vi "Actor Core.vi"(8 "error in":errorcluster, 11 "State in":refnum<class "System Actor.lvclass">) -> (0 "error out":errorcluster, 3 "Actor out":refnum<class "Actor.lvclass">)   [LabVIEW 2014, in "Robot Actor Framework.lvlib" / "System Actor.lvlib" / "System Actor.lvclass"]
doc: "(<B>Filename</B>: Actor Framework.lvlib:Actor.lvclass:Actor Core.vi)\n\nThis override invokes Entry.vi on the initial state, prior to calling the parent Actor Core. Adding this behavior to Actor Core (instead of an override of Pre Launch Init.vi) allows the initial state to launch a nested actor as part of its entry behavior.\n\nReceives messages to the actor, reacts to them, and initiates any error handling that may shut the actor down.\n\nDescendant classes may override this VI to append parallel tasks for the actor to complete while it handles messages. Overrides use the Call Parent Method node."
uses:
  System Actor.lvclass
  <vilib>/ActorFramework/Actor/Actor.lvclass
  System State.ctl
  Command Actor/Command Actor Class/Command State.ctl
  Command Actor/Command Actor Class/Command States.ctl
  Command Processor Actor/Command Processor Actor Class/Command Processor State.ctl
  Command Processor Actor/Command Processor Actor Class/Command Processor States.ctl
  System Actor.lvclass/System Actor.ctl
  Command Processor Actor/States/No Command/No Command.lvclass
  Command Actor/Command Actor Class/Command Actor.lvclass
  Command Processor Actor/Command Processor Actor Class/Command Processor Actor.lvclass
panel:
  out "System Status":T1 {"Command Processor Status"."Commands Behind" scale=0.0..10.0; "Command Processor Status"."Queued Commands" scale=0.0..100.0}
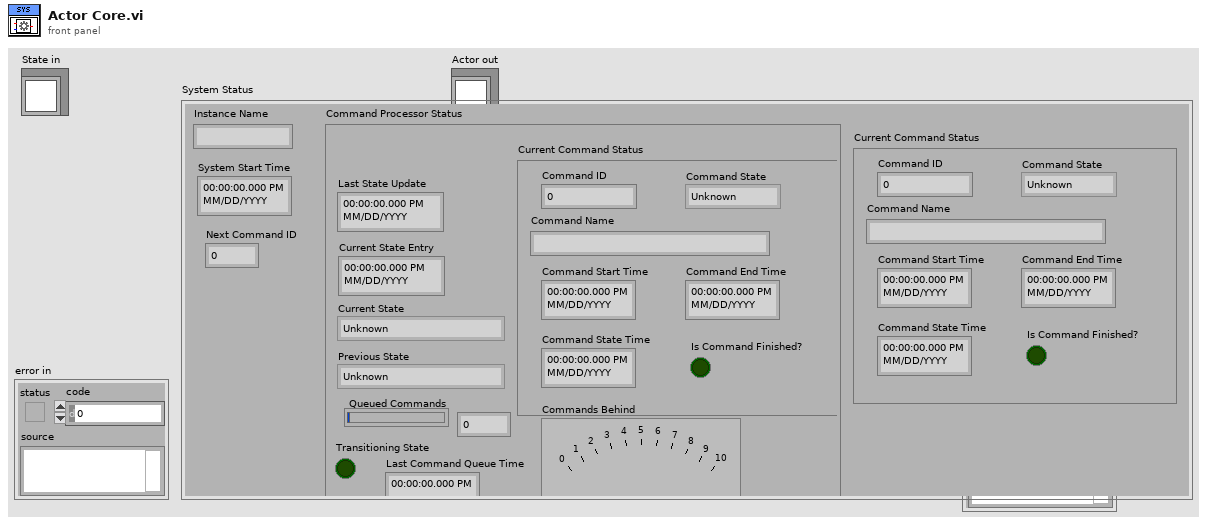
[diagram p1: front panel]
types:
  T1 = typedef "Robot Actor Framework.lvlib/System Actor.lvlib/System Actor.lvclass/System State.ctl" = cluster{"Instance Name":string, "Current Command Status":T2, "System Start Time":timestamp, "Next Command ID":dbl, "Command Processor Status":T4}
  T2 = typedef "Robot Actor Framework.lvlib/Command Actor.lvlib/Command Actor.lvclass/Command State.ctl" = cluster{"Command Name":string, "Command Start Time":timestamp, "Command End Time":timestamp, "Is Command Finished?":bool, "Command ID":u32, "Command State":T3, "Command State Time":timestamp}
  T3 = typedef "Robot Actor Framework.lvlib/Command Actor.lvlib/Command Actor.lvclass/Command States.ctl" = enum16{"Unknown", "Started", "Stopped", "Finished"}
  T4 = typedef "Robot Actor Framework.lvlib/Command Processor Actor.lvlib/Command Processor Actor.lvclass/Command Processor State.ctl" = cluster{"Current State":T5, "Last State Update":timestamp, "Queued Commands":u32, "Current Command Status":T2, "Previous State":T5, "Current State Entry":timestamp, "Transitioning State":bool, "Commands Behind":dbl, "Last Command Queue Time":timestamp}
  T5 = typedef "Robot Actor Framework.lvlib/Command Processor Actor.lvlib/Command Processor Actor.lvclass/Command Processor States.ctl" = enum16{"Unknown", "No Command", "Running Command", "Starting Command", "Stopping Command", "Finishing Command"}
  T6 = enum16{"Critical", "Error", "Warning", "Informational", "Debug"}
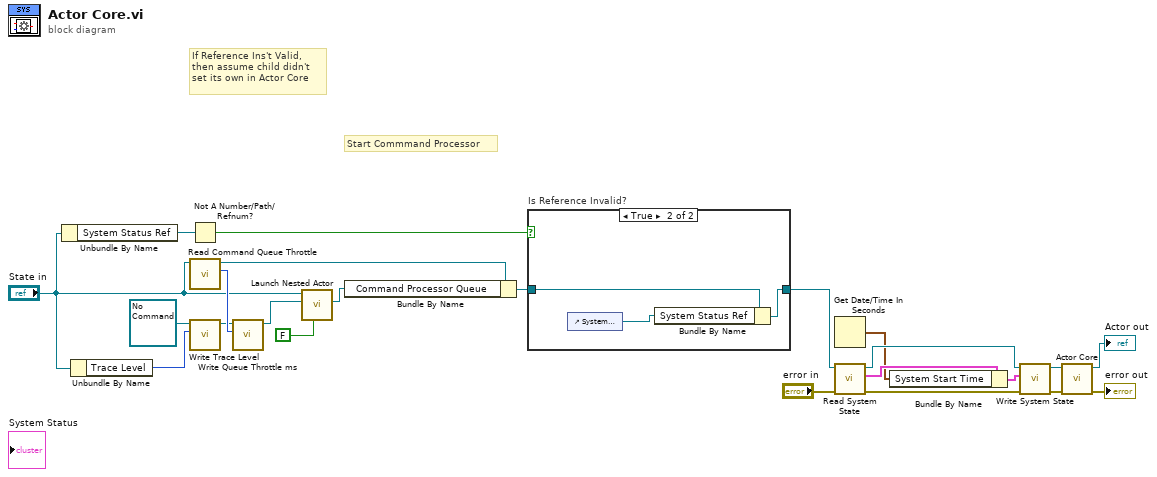
[diagram p0: block diagram]
diagram:
  # "Start Commmand Processor"
  # "If Reference Ins't Valid,\nthen assume child didn't \nset its own in Actor Core"
  n1 = Unbundle By Name("State in") -> ("System Status Ref"=w21:refnum<vi>)
  n2 = Unbundle By Name("State in") -> ("Trace Level"=w1:T6)
  n3 = Not A Number/Path/Refnum?(number/path/refnum=w21) -> (NaN/Path/Refnum?=w20:bool)
  n4 = call-dynamic "Read Command Queue Throttle.vi"("System Actor in"="State in") -> ("Command Queue Throttle ms"=w6:u32, "System Actor out"=w5:refnum<class "System Actor.lvclass">)  [unwired: 8 in, 1 out]
  n5 = call-dynamic "Write Trace Level.vi"("Trace Level"=w1, "Command Processor Actor in"=refnum<class "No Command.lvclass"> refnum ("Robot Actors.lvlib:Command Processor.lvlib:No Command.lvclass")) -> ("Command Processor Actor out"=w2:refnum<class "No Command.lvclass">)  [unwired: 8 in, 1 out]
  n6 = call-dynamic "Write Queue Throttle ms.vi"("Queue Throttle ms"=w6, "Command Processor Actor in"=w2) -> ("Command Processor Actor out"=w7:refnum<class "No Command.lvclass">)  [unwired: 8 in, 1 out]
  n7 = call <vilib>:"Launch Nested Actor.vi"("Open Actor Core front panel? (F)"=FALSE, "Nested Actor"=w7, "Caller Actor in"="State in") -> ("Nested Actor's Enqueuer"=w10:refnum<class "Message Enqueuer.lvclass">)  [unwired: 6 in, 2 out]
  n8 = Bundle By Name(cluster=w5, "Command Processor Queue"=w10) -> (w12:refnum<class "System Actor.lvclass">)
  n9 = case "Is Reference Invalid?" shown="True" w20 {
    tunnel: w12 -> [w24 w27]
    tunnel: [w24 w26] -> w19
    frame False {
    }
    frame True {
      n10 = control-ref of="System Status"() -> (w25:refnum<vi>)
      n11 = Bundle By Name(cluster=w27, "System Status Ref"=w25) -> (w26:refnum<class "System Actor.lvclass">)
    }
  }
  n12 = Get Date/Time In Seconds() -> (seconds since 1Jan1904=w15:timestamp)
  n13 = call-dynamic "Read System State.vi"("error in (no error)"="error in", "System Actor in"=w19) -> ("error out"=w13:errorcluster, "System Status"=w17:T1, "System Actor out"=w18:refnum<class "System Actor.lvclass">)  [unwired: 7 in]
  n14 = Bundle By Name(cluster=w17, "System Start Time"=w15) -> (w16:T1)
  n15 = call-dynamic "Write System State.vi"("error in (no error)"=w13, "System Status"=w16, "System Actor in"=w18) -> ("error out"=w8:errorcluster, "System Actor out"=w9:refnum<class "System Actor.lvclass">)  [unwired: 7 in]
  n16 = call-parent "Actor Core.vi"("error in"=w8, "Actor in"=w9) -> ("error out"=→"error out":errorcluster, "Actor out"=→"Actor out":refnum<class "Actor.lvclass">)  [unwired: 8 in]
